vi "sv_Get Bandedge Frequencies.vi"(9 "octave info":T2={"standard"=enum."ANSI S1.11", "bandwidth"=enum."1 octave", "low band"=0, "high band"=0, "weighting filter"=0, "dB reference"=0.0, "dB On"=FALSE, "unit label"="", "channel name"="", "description"="", "engineering units"=1, "custom label"="", "spectrum type"=enum."magnitude", "spectral density"=FALSE, "filters settled"=FALSE} {"engineering units" items=["custom..."=0, "V"=1, "A"=21, "C"=30, "pC"=31, "s"=32, "-"=29, "Pa"=2, "N"=20, "g"=3, "m/s^2"=4, "m/s"=5, "m"=6, "mm/s"=12, "mm"=13, "micron/s"=14, "micron"=15, "in/s^2"=7, "in/s"=8, "in"=9, "mil/s"=10, "mil"=11, "rad/s^2"=16, "rad/s"=17, "rad"=18, "deg/s^2"=26, "deg/s"=27, "deg"=28, "RPM"=22, "cycle/s^2"=23, "Hz"=24, "cycle"=25, "strain"=19]; "dB reference" format="%.2e"; "weighting filter" items=["Linear", "A-weighting", "B-weighting", "C-weighting", "ITU-R 468-4", "Dolby", "CCITT", "C-message", "Wb", "Wc", "Wd", "We", "Wf", "Wh", "Wj", "Wk", "Wm", "AES17 20 kHz lowpass", "AES17 40 kHz lowpass", "AES17 20 kHz highpass", "AES17 40 kHz highpass"]}, 11 "error in (no error)":errorcluster) -> (6 "bandedge frequencies [Hz]":T1(array[cluster]) {"midband" format="%.2f"; "f high" format="%.2f"; "f low" format="%.2f"}, 15 "error out":errorcluster)   [LabVIEW 2017, in "SoundVib_Octave_2014 standard.lvlib"]
uses:
  <vilib>/addons/Sound and Vibration/svt_Octave/SoundVib_Octave_2014 standard.lvlib
  <vilib>/addons/_NISVFA/_Shared subVIs/Controls/svc_Octave Info.ctl
  <vilib>/addons/_NISVFA/_Shared subVIs/Controls/svc_Octave Standard.ctl
  <vilib>/addons/_NISVFA/_Shared subVIs/Controls/svc_Weighting Filter Text Ring.ctl
  <vilib>/addons/_NISVFA/_Shared subVIs/Controls/svc_Engineering Units Text Ring.ctl
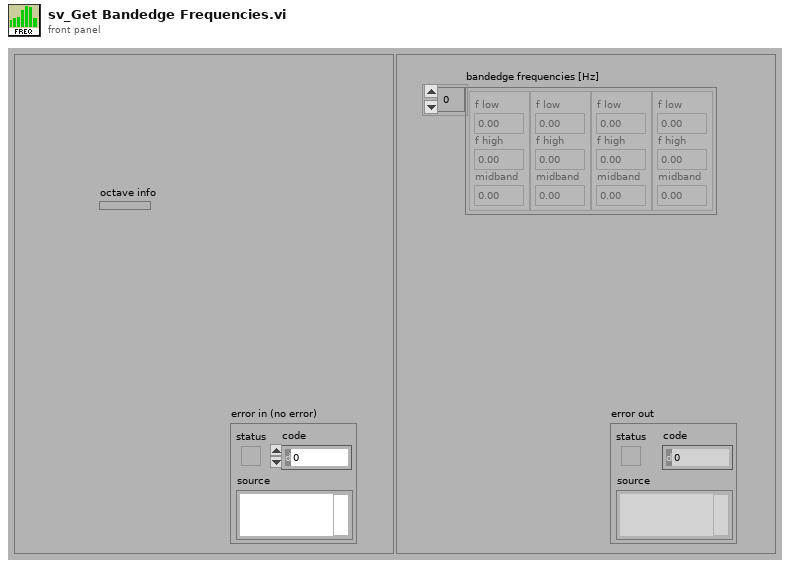
[diagram p1: front panel]
types:
  T1 = cluster{"f low":dbl, "f high":dbl, "midband":dbl}[]
  T2 = typedef "svc_Octave Info.ctl" = cluster{"standard":T3, "bandwidth":enum16{"1 octave", "1/3 octave", "1/6 octave", "1/12 octave", "1/24 octave"}, "low band":i32, "high band":i32, "weighting filter":T4, "dB reference":dbl, "dB On":bool, "unit label":string, "channel name":string, "description":string, "engineering units":T5, "custom label":string, "spectrum type":enum16{"power", "magnitude"}, "spectral density":bool, "filters settled":bool}
  T3 = typedef "svc_Octave Standard.ctl" = enum16{"ANSI S1.11", "IEC 61260"}
  T4 = typedef "svc_Weighting Filter Text Ring.ctl" = u16
  T5 = typedef "svc_Engineering Units Text Ring.ctl" = u16
  T6 = enum16{"1 octave", "1/3 octave", "1/6 octave", "1/12 octave", "1/24 octave"}
  T7 = cluster{"f low":dbl, "f high":dbl, "midband frequency [Hz]":dbl}
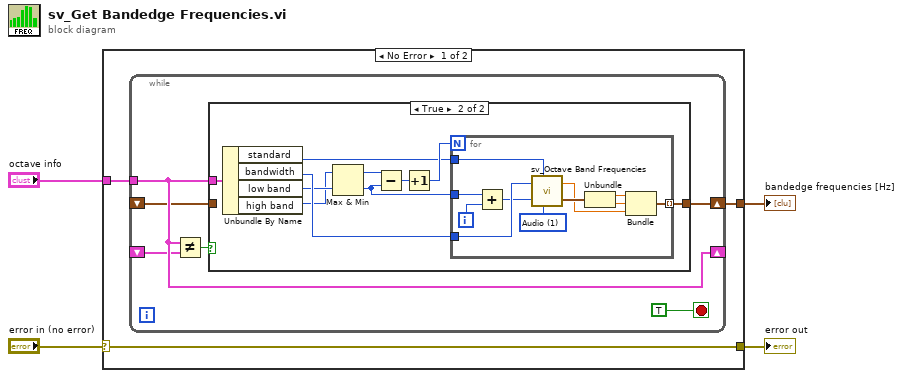
[diagram p0: block diagram]
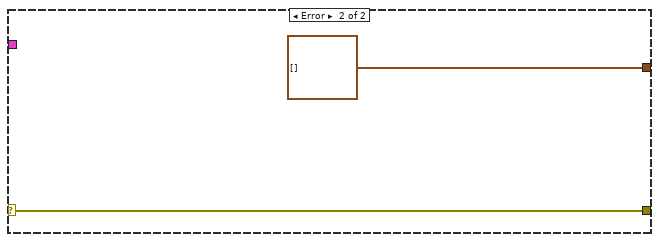
[diagram p3: hidden frame]
diagram:
  n1 = case shown="No Error" "error in (no error)" {
    selector: "error in (no error)" -> [w5 w37]
    tunnel: [w5 w37] -> w3
    tunnel: [w6 T1 [] ("bandedge frequencies [Hz]")] -> w2
    tunnel: "octave info" -> [w7 _]
    frame No Error {
      n2 = while {
        shift-left: _ -> [w8]
        shift-right: [w13] -> w6
        shift-left: _ -> [w11]
        shift-right: [w12] -> _
        tunnel: w7 -> [w12]
        stop <- TRUE stop-if-true
        n3 = Not Equal?(x=w12, y=w11) -> (x != y?=w10:bool)
        n4 = case shown="True" w10 {
          tunnel: [w14 w21] -> w13
          tunnel: w12 -> [_ w15]
          tunnel: w8 -> [w14 _]
          frame False {
          }
          frame True {
            n5 = Unbundle By Name(w15) -> ("standard"=w19:T3, "bandwidth"=w18:T6, "low band"=w17:i32, "high band"=w16:i32)
            n6 = Max & Min(x=w16, y=w17) -> (max(x,y)=w23:i32, min(x,y)=w24:i32)
            n7 = Subtract(x=w23, y=w24) -> (x-y=w22:i32)
            n8 = Increment(x=w22) -> (x+1=w20:i32)
            n9 = for {
              N: w20 -> [_]
              tunnel: w24 -> [w35]
              tunnel: w18 -> [w27]
              tunnel: [w29] -> w21 mode=indexing
              tunnel: w19 -> [w28]
              i -> [w34]
              w33 = u16 1 items=["Infrasonic", "Audio", "Ultrasonic"] ("Frequency range")
              n10 = Add(x=w35, y=w34) -> (x+y=w26:i32)
              n11 = call <vilib>:"sv_Octave Band Frequencies.vi"("octave band selector"=w26, "reference frequency range"=w33, "bandwidth"=w27, "standard"=w28) -> ("bandedge frequencies [Hz]"=w32:cluster{"f low":dbl, "f high":dbl}, "midband frequency [Hz]"=w25:dbl)  [unwired: 2 out]
              n12 = Unbundle(w32) -> ("f low"=w31:dbl, "f high"=w30:dbl)
              n13 = Bundle("f low"=w31, "f high"=w30, "midband frequency [Hz]"=w25) -> (w29:T7)  [unwired: 1 in]
            }
          }
        }
      }
    }
    frame Error {
      (unwired) string[] [] ("nominal frequencies (string)")
    }
  }
  "error out" <- w3
  "bandedge frequencies [Hz]" <- w2
